vi "Send Message.vi"(8 "error in (no error)":errorcluster, 10 "Message In":refnum<class "Message.lvclass">, 11 "Messenger in":refnum<class "Messenger.lvclass">) -> (0 "error out":errorcluster)   [LabVIEW 2015, in "Messenger.lvclass"]
uses:
  Messenger.lvclass
  Message/Message.lvclass
  Messenger.lvclass/Messenger.ctl
  Message/Message.lvclass/Message.ctl
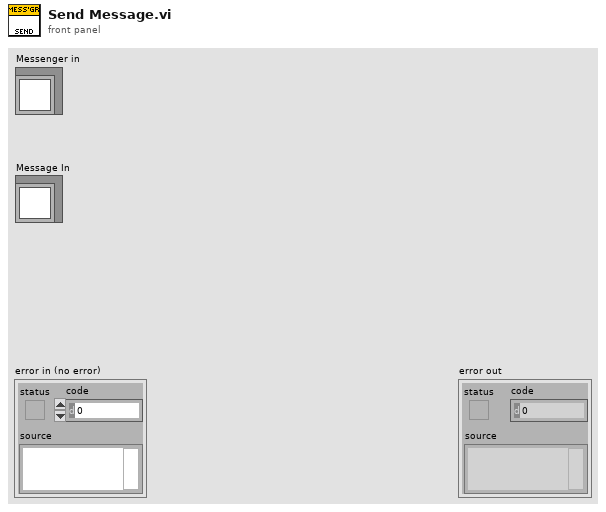
[diagram p1: front panel]
types:
  T1 = typedef "usereventprio.ctl" = enum32{"high priority", "normal priority"}
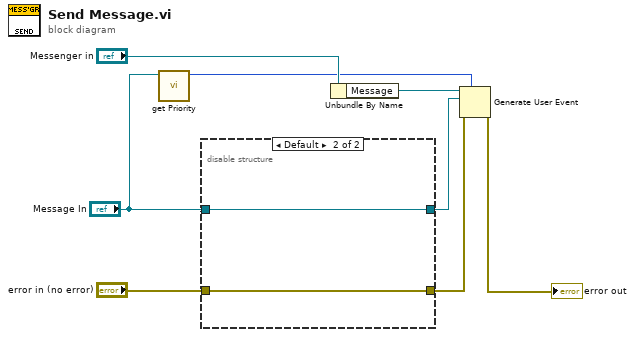
[diagram p0: block diagram]
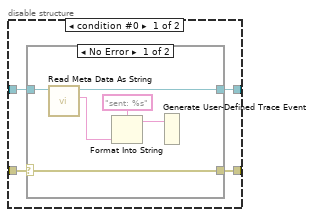
[diagram p2: hidden frame]
diagram:
  n1 = call "get Priority.vi"("Message in"="Message In") -> ("user event priority"=w2:T1)  [unwired: 10 in]
  n2 = disable-structure shown="Default" {
    disable-tunnel: "Message In" -> [w12 w22]
    disable-tunnel: [w11 w22] -> w5
    disable-tunnel: "error in (no error)" -> [w10 w21]
    disable-tunnel: [w9 w21] -> w3
    frame condition #0 {
      n3 = case shown="No Error" w10 {
        selector: w10 -> [w16 w20]
        tunnel: w12 -> [w15 w19]
        tunnel: [w14 w19] -> w11
        tunnel: [w16 w20] -> w9
        frame No Error {
          n4 = call-dynamic "Read Meta Data As String.vi"("Message in"=w15) -> ("Meta Data"=w13:string, "Message out"=w14:refnum<class "Message.lvclass">)  [unwired: 8 in, 1 out]
          n5 = Format Into String(format string="sent: %s", w13) -> (resulting string=w18:string)  [unwired: 2 in, 1 out]
          n6 = Generate User-Defined Trace Event(2:w18) -> ()  [unwired: 1 in]
        }
        frame Error {
        }
      }
    }
    frame condition #1 (active) {
    }
  }
  n7 = Unbundle By Name("Messenger in") -> ("Message"=w7:refnum<user-event>)
  n8 = Generate User Event(priority (normal)=w2, user event=w7, event data cluster=w5, error in=w3) -> (error out=→"error out":errorcluster)  [unwired: 1 out]
